vi "Count.vi"(3 "IMsgPackContainer in":refnum<class "IMsgPackContainer.lvclass">) -> (1 "Count":u64)   [LabVIEW 2020, in "MessagePack.lvlib" / "IMsgPackContainer.lvclass"]
uses:
  IMsgPackContainer.lvclass
panel:
  out "IMsgPackContainer out":refnum<class "IMsgPackContainer.lvclass">
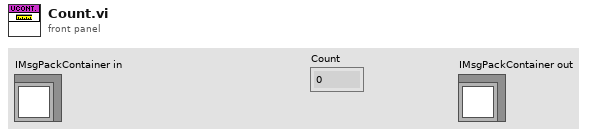
[diagram p1: front panel]
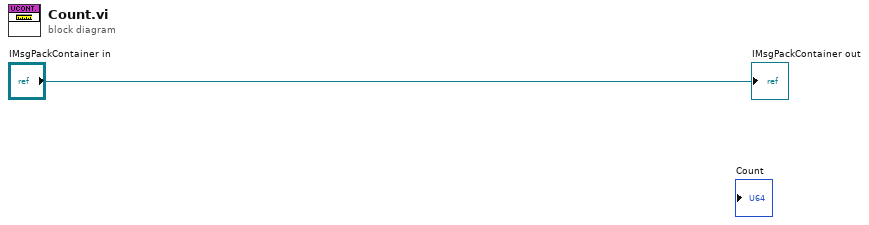
[diagram p0: block diagram]
diagram:
  "IMsgPackContainer out" <- "IMsgPackContainer in"
